vi "Dock or Undock.vi"(8 "error in (no error)":errorcluster, 10 "Action":T1, 11 "Assert Startup UI in":refnum<class "Assert Startup UI.lvclass">) -> (0 "error out":errorcluster, 3 "Assert Startup UI out":refnum<class "Assert Startup UI.lvclass">)   [LabVIEW 2016, in "Assert API Components.lvlib" / "Assert Startup UI.lvlib" / "Assert Startup UI.lvclass"]
uses:
  Assert Startup UI.lvclass
  System Tray Docking Actions.ctl
  Assert Startup UI.lvclass/Assert Startup UI.ctl
  System Tray/NotifyIcon.lvclass
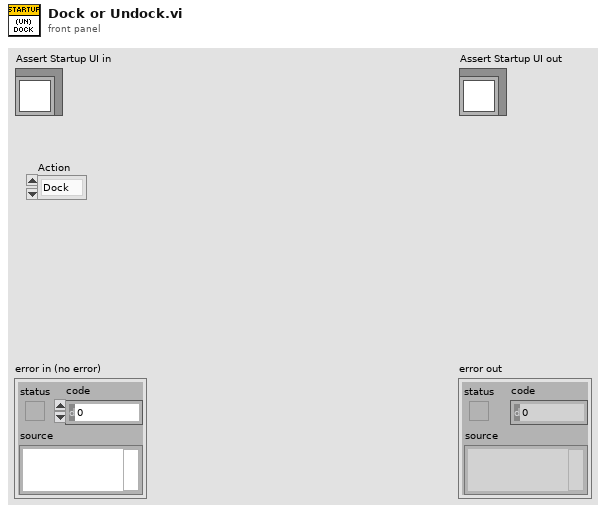
[diagram p1: front panel]
types:
  T1 = typedef "Assert API Components.lvlib/Assert Startup UI.lvlib/Assert Startup UI.lvclass/System Tray Docking Actions.ctl" = enum16{"Dock", "Undock"}
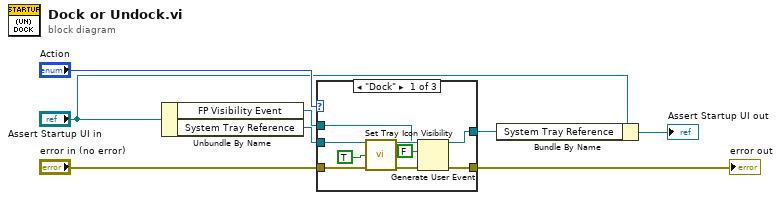
[diagram p0: block diagram]
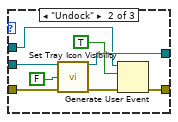
[diagram p2: hidden frame]
diagram:
  n1 = Unbundle By Name("Assert Startup UI in") -> ("FP Visibility Event"=w1:refnum<user-event>, "System Tray Reference"=w6:refnum<class "NotifyIcon.lvclass">)
  n2 = case shown="\"Dock\"" "Action" {
    tunnel: w6 -> [w16 w24 w26]
    tunnel: [w15 w23 w26] -> w4
    tunnel: "error in (no error)" -> [w14 w22 w25]
    tunnel: [w11 w19 w25] -> w2
    tunnel: w1 -> [w10 w18 _]
    frame "Dock" {
      n3 = call "Set Tray Icon Visibility.vi"("NotifyIcon in"=w16, "Show Tray Icon"=TRUE, "error in (no error)"=w14) -> ("NotifyIcon out"=w15:refnum<class "NotifyIcon.lvclass">, "error out"=w13:errorcluster)  [unwired: 11 out]
      n4 = Generate User Event(user event=w10, event data cluster=FALSE ("event data"), error in=w13) -> (error out=w11:errorcluster)  [unwired: 1 in, 1 out]
    }
    frame "Undock" {
      n5 = call "Set Tray Icon Visibility.vi"("NotifyIcon in"=w24, "Show Tray Icon"=FALSE, "error in (no error)"=w22) -> ("NotifyIcon out"=w23:refnum<class "NotifyIcon.lvclass">, "error out"=w21:errorcluster)  [unwired: 11 out]
      n6 = Generate User Event(user event=w18, event data cluster=TRUE ("event data"), error in=w21) -> (error out=w19:errorcluster)  [unwired: 1 in, 1 out]
    }
    frame Default {
    }
  }
  "error out" <- w2
  n7 = Bundle By Name(cluster="Assert Startup UI in", "System Tray Reference"=w4) -> (→"Assert Startup UI out":refnum<class "Assert Startup UI.lvclass">)
